vi "请求注册.vi"(8 "error in (no error)":errorcluster caption="错误输入（无错误）", 10 "数据采集 输入":refnum<class "数据采集.lvclass"> caption="DNL_LabVIEW Object in", 11 "数据显示 输入":refnum<class "数据显示.lvclass"> caption="DNL_LabVIEW Object in") -> (0 "error out":errorcluster caption="错误输出", 2 "数据采集 输出":refnum<class "数据采集.lvclass"> caption="DNL_LabVIEW Object out", 3 "数据显示 输出":refnum<class "数据显示.lvclass"> caption="DNL_LabVIEW Object out")   [LabVIEW 2013, in "数据显示.lvclass"]
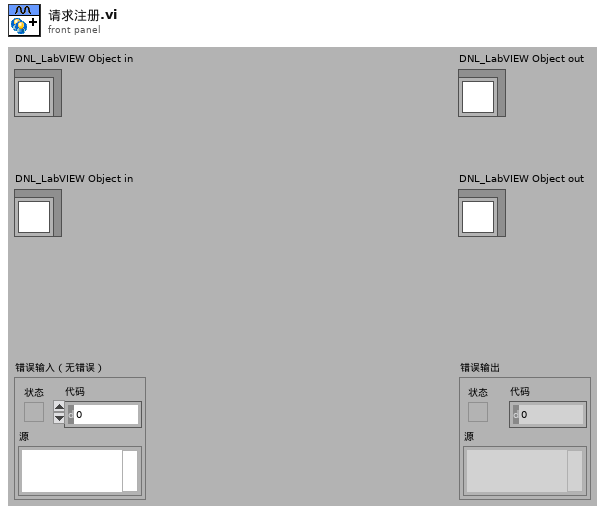
[diagram p1: front panel]
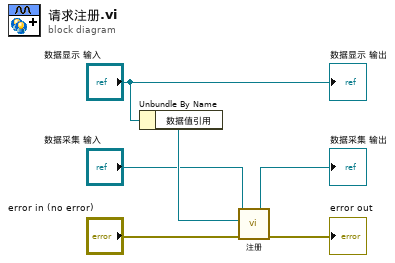
[diagram p0: block diagram]
diagram:
  n1 = Unbundle By Name("数据显示 输入") -> ("数据值引用"=w4:refnum<data-value>)
  n2 = call-dynamic "注册.vi"("error in (no error)"="error in (no error)", "数据值引用"=w4, "数据采集 输入"="数据采集 输入") -> ("error out"=→"error out":errorcluster, "数据采集 输出"=→"数据采集 输出":refnum<class "数据采集.lvclass">)  [unwired: 7 in]
  "数据显示 输出" <- "数据显示 输入"
